vi "fft_fit.vi"(8 "error in (no error)":errorcluster, 10 "LR":waveform(dbl), 11 "Refnum in":refnum<k35>) -> (0 "error out":errorcluster, 2 "psd":cluster{dbl[], dbl[]}, 3 "Refnum out":refnum<k35>)   [LabVIEW 2026]
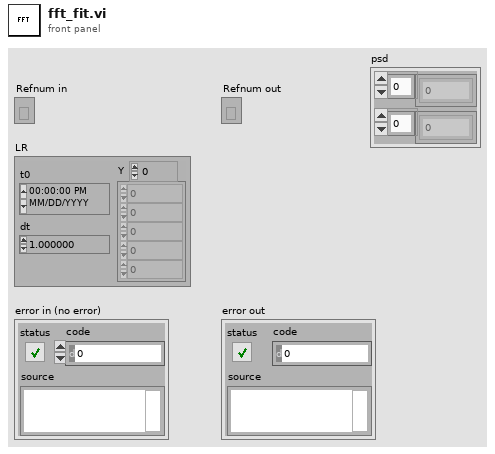
[diagram p1: front panel]
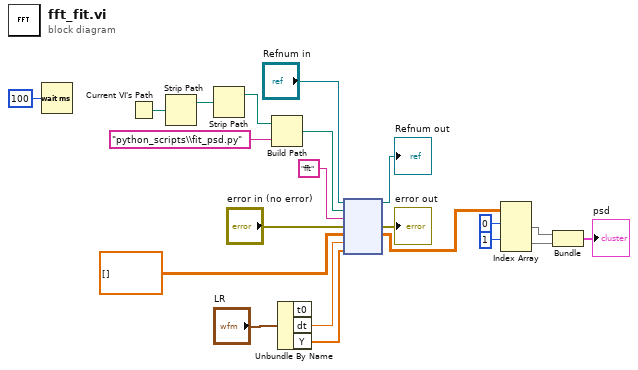
[diagram p0: block diagram]
diagram:
  n1 = Wait (ms)(milliseconds to wait=u32 100) -> ()  [unwired: 1 out]
  n2 = Current VI's Path() -> (path=w12:path)
  n3 = Strip Path(path=w12) -> (stripped path=w9:path)  [unwired: 1 out]
  n4 = Strip Path(path=w9) -> (stripped path=w8:path)  [unwired: 1 out]
  n5 = Build Path(base path=w8, name or relative path="python_scripts\\fit_psd.py") -> (appended path=w11:path)
  n6 = Unbundle By Name("LR") -> ("dt"=w10:dbl, "Y"=w21:dbl[])  [unwired: 1 out]
  n7 = node("Refnum in", w11, "fft" ("function name"), "error in (no error)", dbl[][] [], w10, w21) -> (→"Refnum out":refnum<k35>, →"error out":errorcluster, w7:dbl[][])  [unwired: 2 in, 2 out]
  n8 = Index Array(array=w7, index (row) #1=0 ("index (row)"), index (row) #2=1 ("index (row)")) -> (element #1=w4:dbl[], element #2=w3:dbl[])  [unwired: 2 in]
  n9 = Bundle(w4, w3) -> (→"psd":cluster{dbl[], dbl[]})  [unwired: 1 in]
